vi "Read Lock Publication Msg.vi"(11 "IModel in":refnum<class "IModel.lvclass">) -> (2 "Pre-Addressed Lock Msg":refnum<class "Lock Publication Msg.lvclass">)   [LabVIEW 2015, in "IModel.lvlib" / "IModel.lvclass"]
uses:
  IModel.lvclass
  IMediator/IMediator Messages/Lock Publication Msg/Lock Publication Msg.lvclass
  IModel.lvclass/IModel.ctl
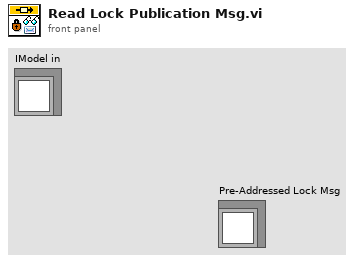
[diagram p1: front panel]
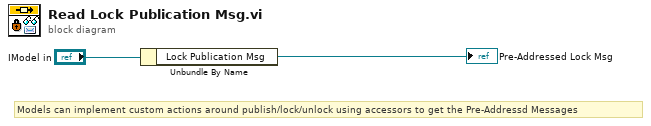
[diagram p0: block diagram]
diagram:
  # "Models can implement custom actions around publish/lock/unlock using accessors to get the Pre-Addressd Messages"
  n1 = Unbundle By Name("IModel in") -> ("Lock Publication Msg"=→"Pre-Addressed Lock Msg":refnum<class "Lock Publication Msg.lvclass">)
